vi "Edit_Raw_DF_Header.vi"(0 "Selected files":path[](array[path])) -> ()   [LabVIEW 2013]
uses:
  Controls/File_Selector_Type.ctl
panel:
  in  "Variable names to add by hand":string[](array[string])
  in  "Variable values to add by hand":string[](array[string])
  out "No of Unfound files":i32
  out "Unfound Files":path[](array[path])
  out "File Number":i32
  out "Current case":string
  out "Currently Editting":path
  out "Summary values":string[](array[string])
  in  "New Variable values":string[](array[string])
  in  "Setup Information":i32[](listbox)
  in  "Variable names to Edit":string[](array[string])
  in  "OK":bool
  out "No of Files":i32
  in  "Previous Choice":path
  in  "Search String":string
  in  "At Dialog Prompt for Editting Raw data files":T1
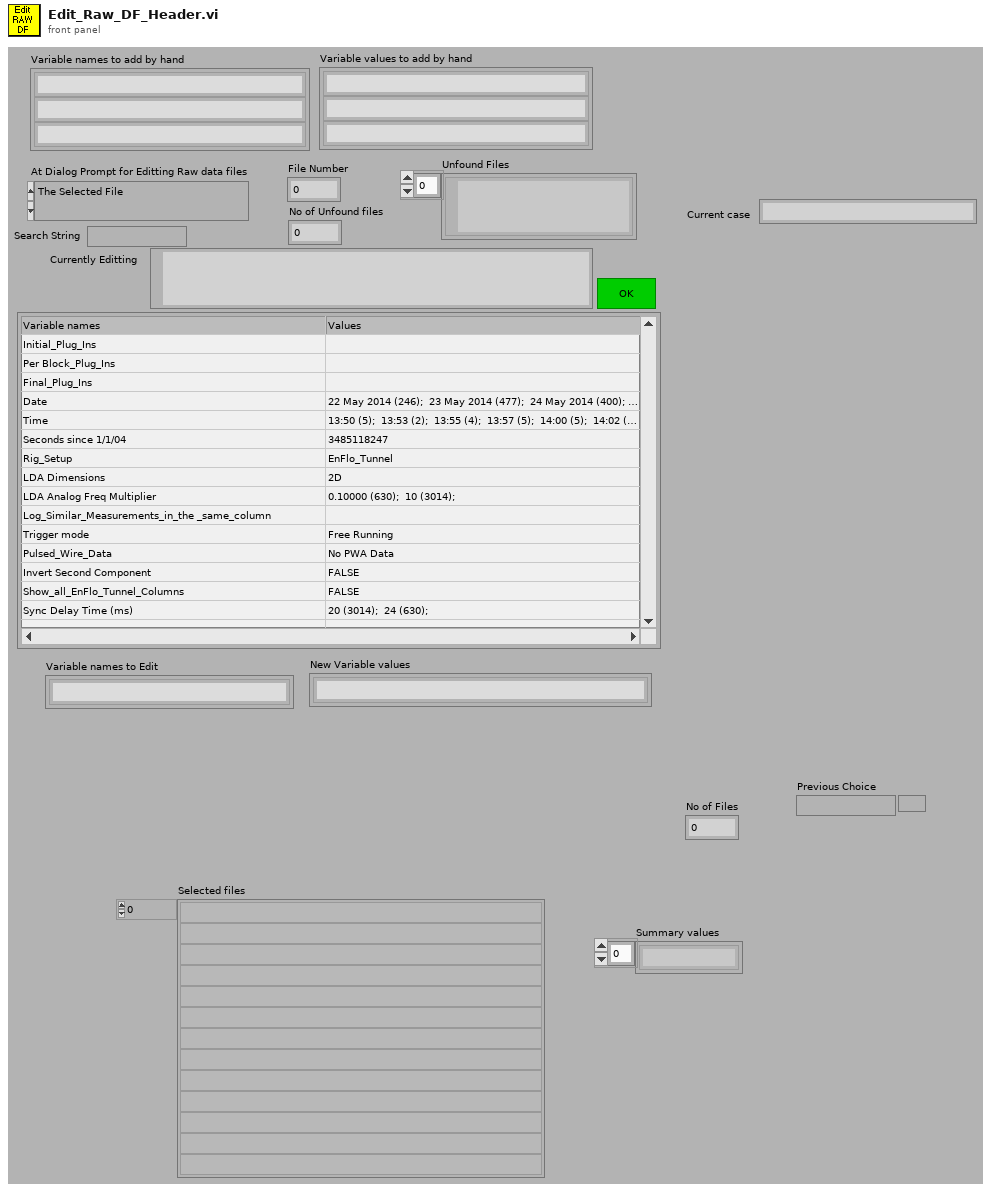
[diagram p1: front panel]
types:
  T1 = typedef "File_Selector_Type.ctl" = enum16{"The Selected File", "The Selected Folder", "Files containing the search string in the selected folder", "All files listed in selected file"}
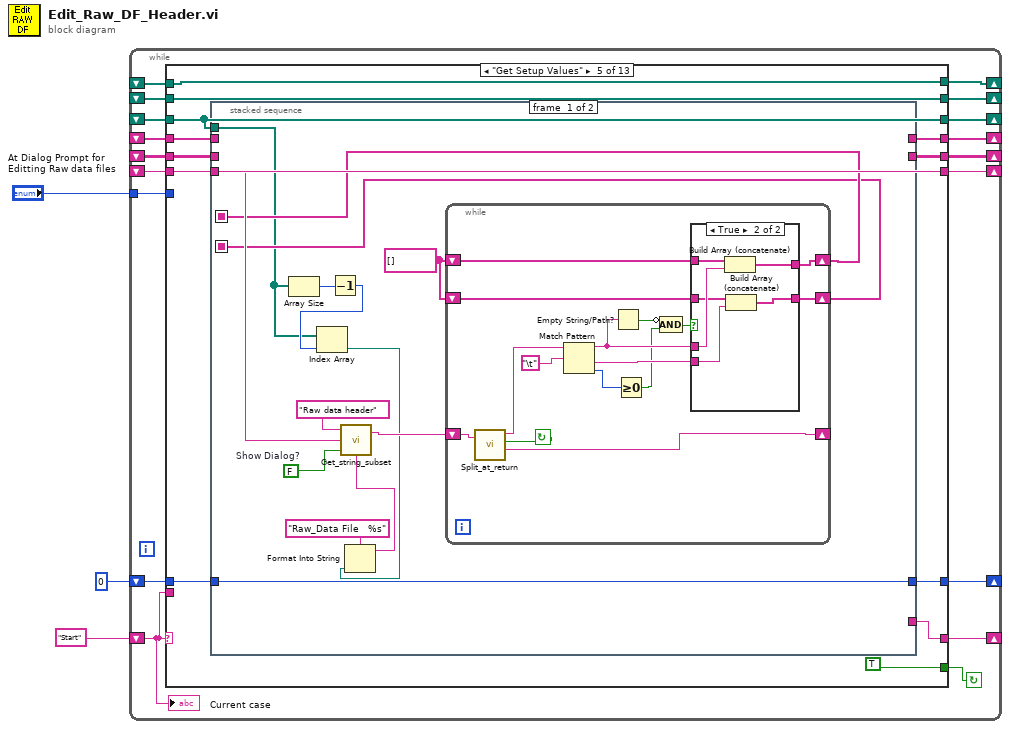
[diagram p0: block diagram]
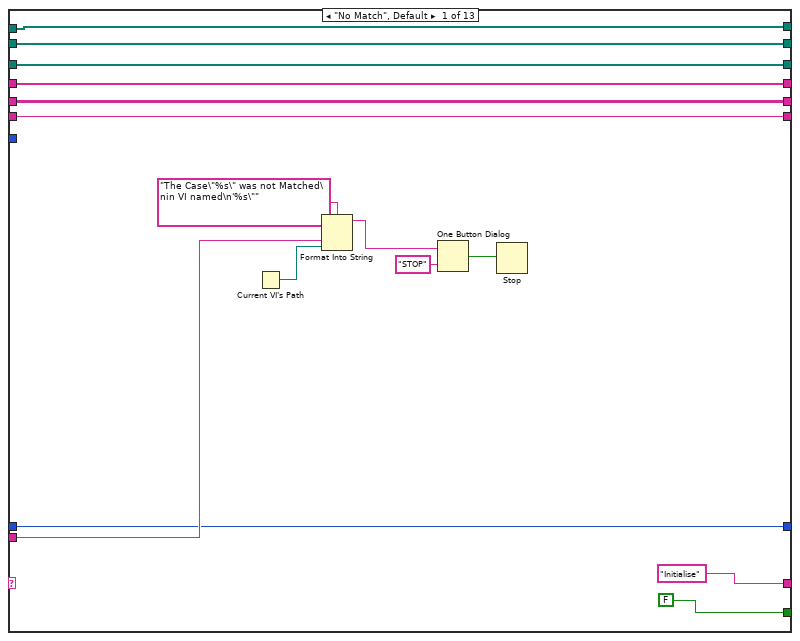
[diagram p2: hidden frame]
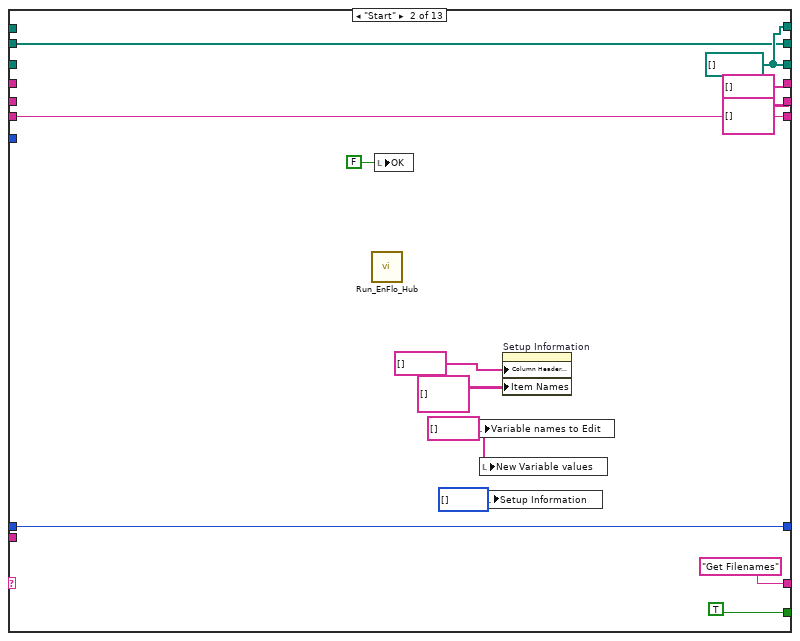
[diagram p3: hidden frame]
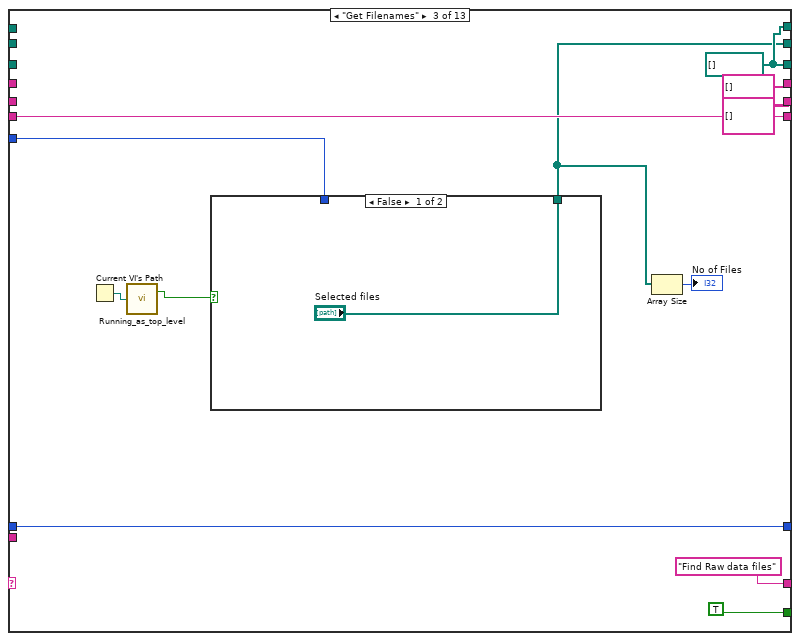
[diagram p4: hidden frame]
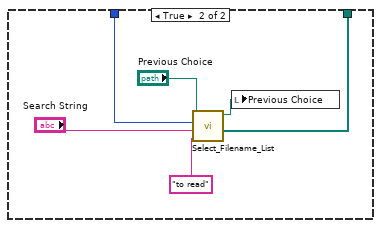
[diagram p5: hidden frame]
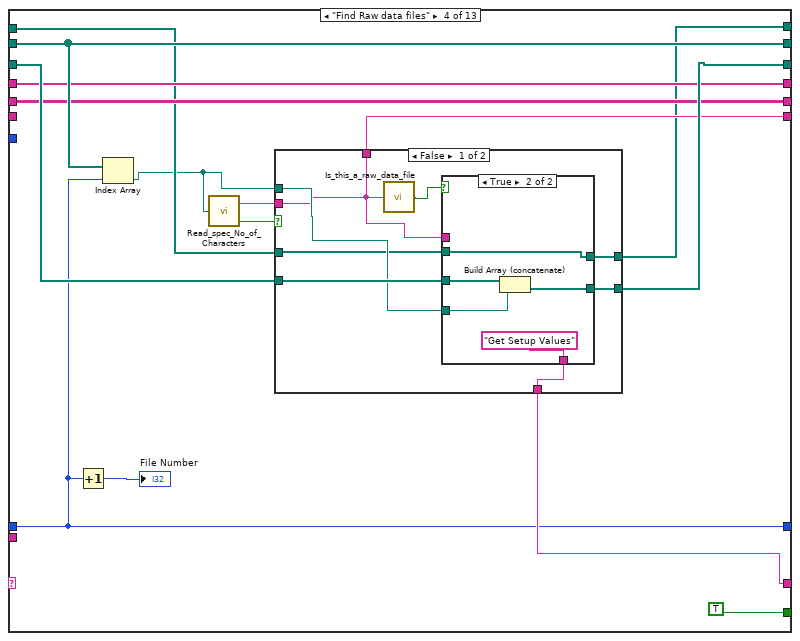
[diagram p6: hidden frame]
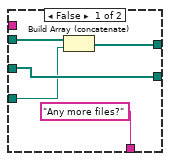
[diagram p7: hidden frame]
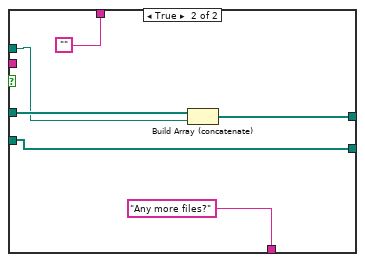
[diagram p8: hidden frame]
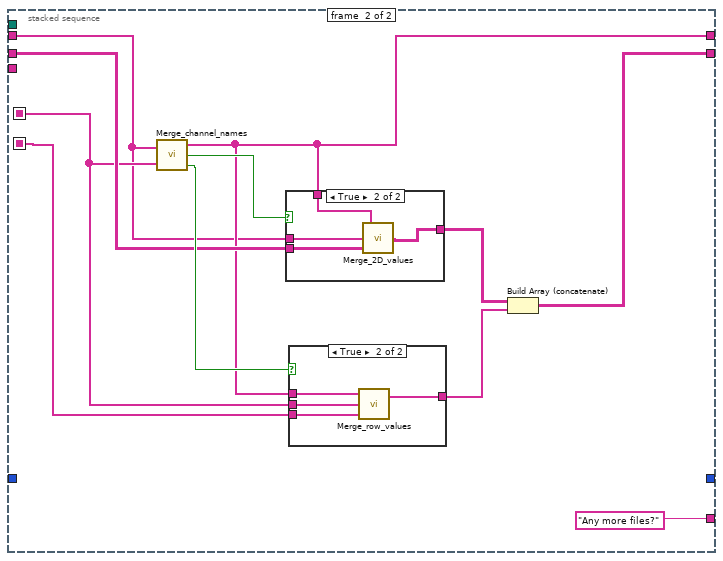
[diagram p10: hidden frame]
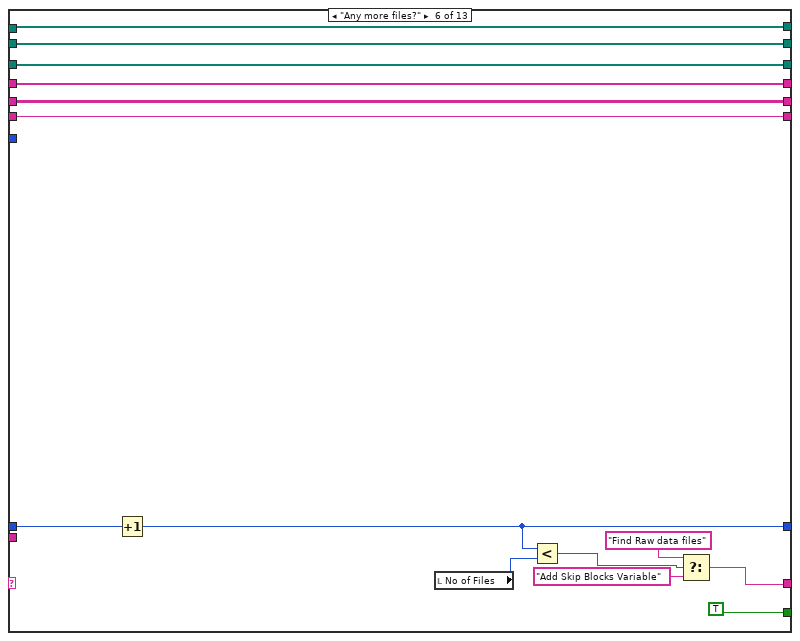
[diagram p13: hidden frame]
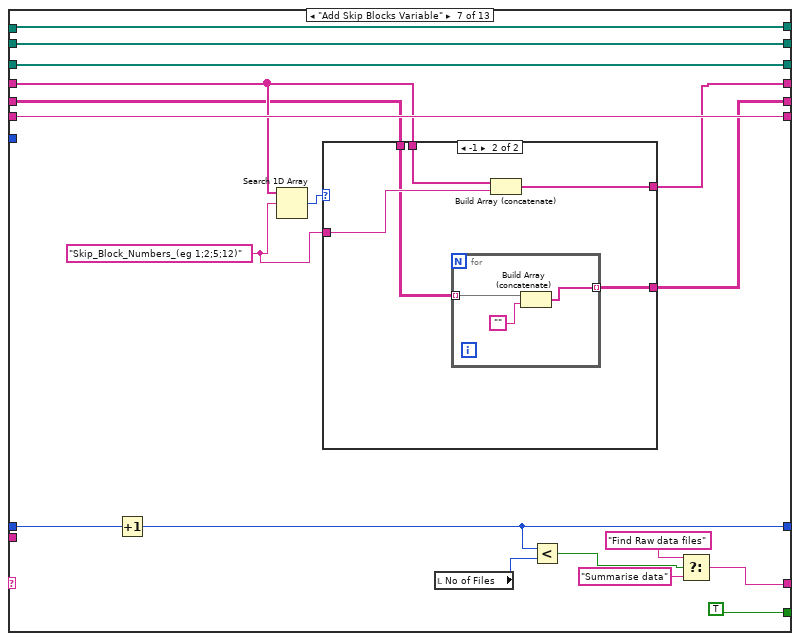
[diagram p14: hidden frame]
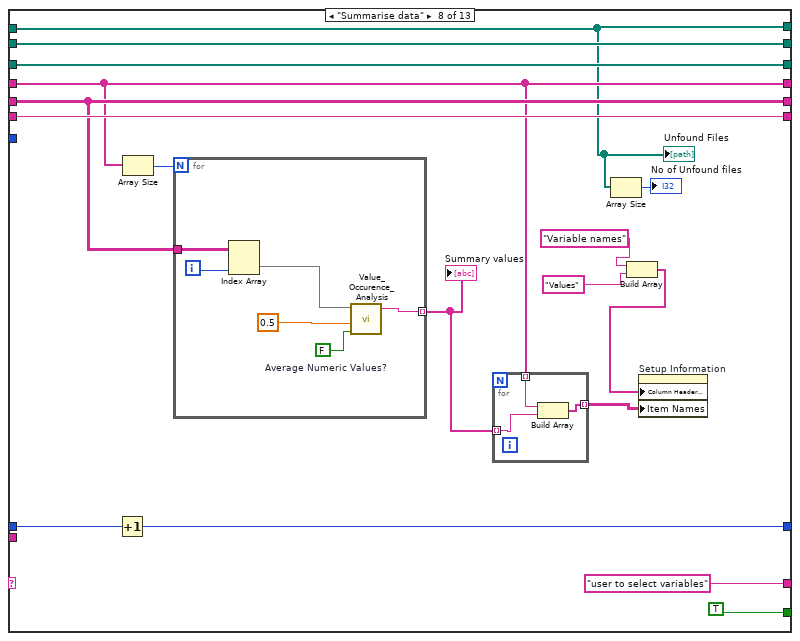
[diagram p16: hidden frame]
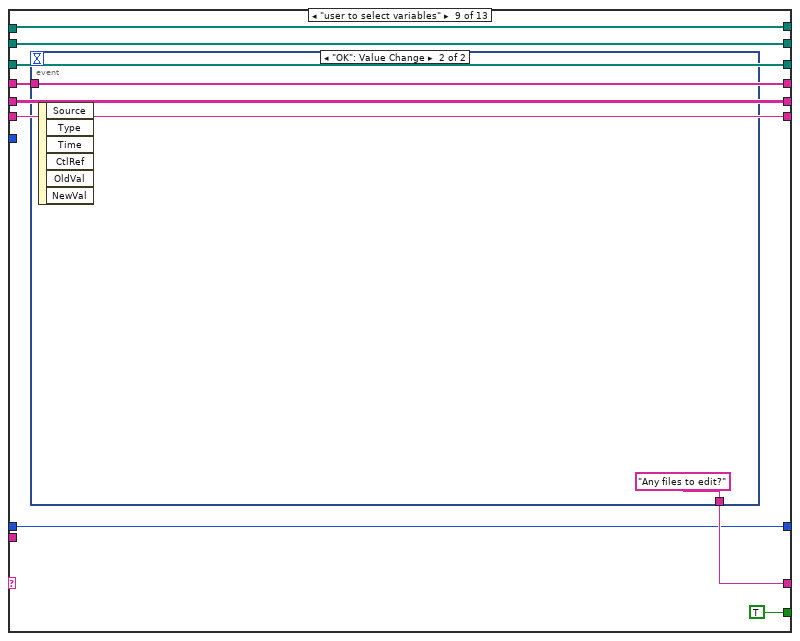
[diagram p17: hidden frame]
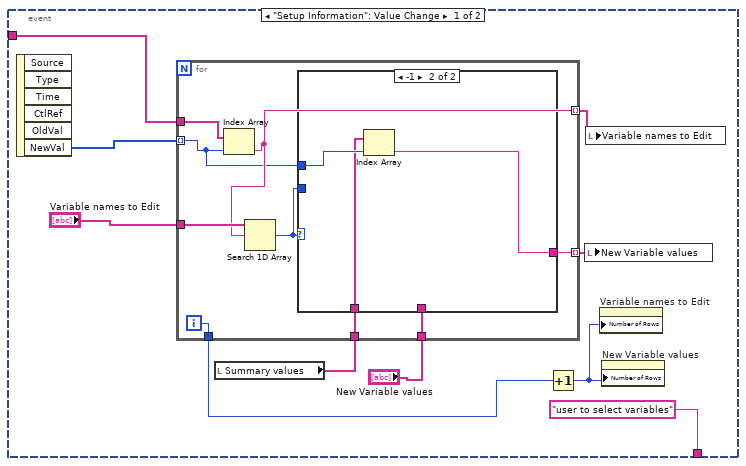
[diagram p18: hidden frame]
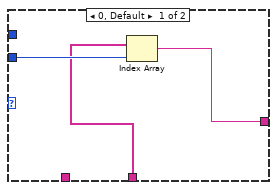
[diagram p19: hidden frame]
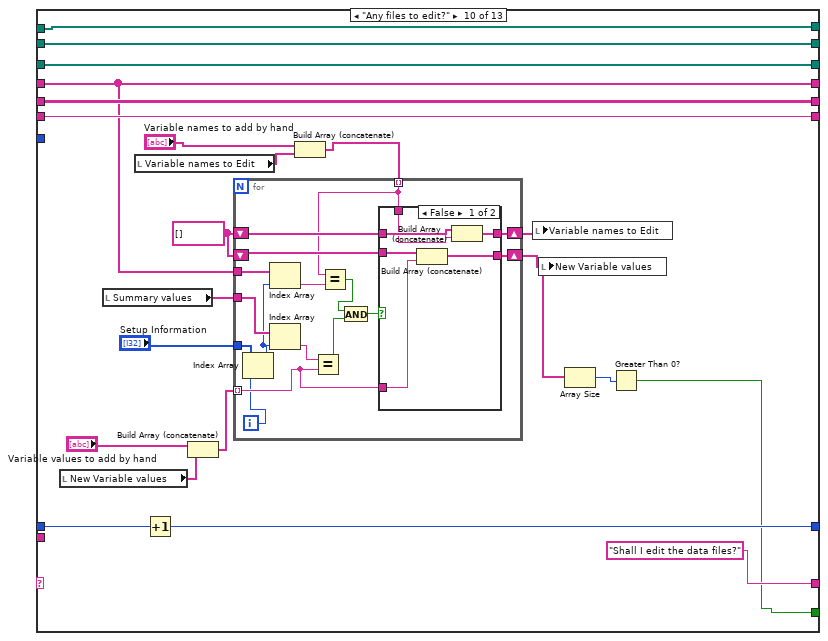
[diagram p20: hidden frame]
diagram:
  n1 = while {
    shift-left: "Start" -> [w19]
    shift-right: [w20] -> _
    shift-right: [w17] -> _
    shift-left: _ -> [w18]
    tunnel: "At Dialog Prompt for Editting Raw data files" -> [w16]
    shift-right: [w7] -> _
    shift-left: 0 -> [w13]
    shift-right: [w15] -> _
    shift-left: _ -> [w14]
    shift-right: [w12] -> _
    shift-left: _ -> [w11]
    shift-right: [w9] -> _
    shift-left: _ -> [w10]
    shift-right: [w8] -> _
    shift-left: _ -> [w6]
    shift-right: [w4] -> _
    shift-left: _ -> [w5]
    stop <- w21 continue-if-true
    n2 = case shown="\"Get Setup Values\"" w19 {
      tunnel: [FALSE TRUE TRUE TRUE TRUE TRUE TRUE TRUE TRUE w289 w328 TRUE ("T button?") FALSE ("T button?")] -> w21
      tunnel: ["Initialise" "Get Filenames" "Find Raw data files" w76 w115 w183 w202 "user to select variables" w248 "Shall I edit the data files?" "Edit Raw data files" "End" "End"] -> w20
      tunnel: w19 -> [w31 _ _ _ _ _ _ _ _ _ _ _ _]
      tunnel: w18 -> [w28 w37 _ w80 w118 w190 w208 w235 w254 w302 w338 w349 w364]
      tunnel: [w28 w37 w50 w80 w118 w190 w208 w235 w254 w302 w338 w349 w364] -> w17
      tunnel: w16 -> [_ _ w60 _ _ _ _ _ _ _ _ _ _]
      tunnel: w14 -> [w27 _ _ w82 w108 w182 w201 w232 w253 w299 w332 w342 w358]
      tunnel: [w27 w38 w53 w81 w108 w182 w201 w232 w253 w299 w332 w342 w358] -> w15
      tunnel: w13 -> [w23 w44 w54 w75 w117 w188 w207 w234 w247 w301 w333 w344 w359]
      tunnel: [w26 string[] [] ("Merged Channels") string[] [] ("Merged Channels") w79 w113 w178 w196 w228 w249 w287 w335 w346 w361] -> w12
      tunnel: w11 -> [w26 _ _ w79 w110 w178 w197 w228 w249 w287 w335 w346 w361]
      tunnel: w10 -> [w25 _ _ w78 w112 w189 w193 w230 w251 w297 w336 w347 w362]
      tunnel: [w25 string[][] [] string[][] [] w78 w111 w189 w192 w230 w251 w297 w336 w347 w362] -> w9
      tunnel: [w24 w47 w57 w77 w114 w181 w200 w231 w252 w298 w337 w348 w363] -> w8
      tunnel: [w23 w44 w54 w75 w116 w187 w206 w233 w247 w300 w333 w344 w359] -> w7
      tunnel: w6 -> [w24 w47 w57 _ w114 w181 w200 w231 w252 w298 w337 w348 w363]
      tunnel: w5 -> [w22 _ _ w74 w109 w179 w198 w221 w246 w288 w327 w339 w354]
      tunnel: [w22 w38 w53 w73 w109 w179 w198 w221 w246 w288 w327 w339 w354] -> w4
      frame "No Match", Default {
        n3 = Current VI's Path() -> (path=w30:path)
        n4 = Format Into String(format string="The Case\"%s\" was not Matched\nin VI named\n'%s\"" ("Format String"), w31, w30) -> (resulting string=w34:string)  [unwired: 2 in, 1 out]
        n5 = One Button Dialog(message=w34, button name ("OK")="STOP") -> (true=w32:bool)
        n6 = Stop(stop? (T)=w32) -> ()
      }
      frame "Start" {
        w43 = string[] [] ("Variable names to Edit")
        w38 = path[] []
        n7 = call "Run_EnFlo_Hub.vi"() -> ()  [unwired: 8 out]
        n8 = local write "OK"(FALSE ("OK")) -> ()
        n9 = local write "Variable names to Edit"(w43) -> ()
        n10 = local write "New Variable values"(w43) -> ()
        n11 = local write "Setup Information"(i32[] [] ("Setup Information")) -> ()
        n12 = property on="Setup Information" class="MCListbox (strict)"("Column Header Strings[]"=string[] [] ("Column Header Strings"), "Item Names"=string[][] []) -> ()  [unwired: 2 in, 2 out]
      }
      frame "Get Filenames" {
        w53 = path[] []
        n13 = Current VI's Path() -> (path=w52:path)
        n14 = call "Running_as_top_level.vi"("Vi path name"=w52) -> ("Top Level"=w51:bool)  [unwired: 1 out]
        n15 = case shown="False" w51 {
          tunnel: w60 -> [_ w68]
          tunnel: ["Selected files" w63] -> w50
          frame False {
          }
          frame True {
            n16 = call "Select_Filename_List.vi"("File Type"="to read", "Search String"="Search String", "At Dialog Prompt Post Process"=w68, "Previous Choice"="Previous Choice") -> ("Selected files"=w63:path[], "Choosen path"=w64:path)  [unwired: 1 in, 2 out]
            n17 = local write "Previous Choice"(w64) -> ()
          }
        }
        n18 = Array Size(array=w50) -> (size(s)=→"No of Files":i32)
      }
      frame "Find Raw data files" {
        n19 = Increment(x=w75) -> (x+1=→"File Number":i32)
        n20 = Index Array(array=w80, index=w75) -> (element=w72:path)
        n21 = call "Read_spec_No_of_Characters.vi"("Filename"=w72) -> ("character string"=w70:string, "Error?"=w71:bool)
        n22 = case shown="False" w71 {
          tunnel: w82 -> [w91 w107]
          tunnel: [w90 w107] -> w81
          tunnel: w72 -> [w88 w103]
          tunnel: [w84 ""] -> w77
          tunnel: [w87 "Any more files?"] -> w76
          tunnel: w74 -> [w86 w104]
          tunnel: [w85 w102] -> w73
          tunnel: w70 -> [w84 _]
          frame False {
            n23 = call "Is_this_a_raw_data_file.vi"("character string"=w84) -> ("Raw Dat File?"=w89:bool)  [unwired: 2 out]
            n24 = case shown="True" w89 {
              tunnel: w91 -> [w96 w101]
              tunnel: w88 -> [w92 w100]
              tunnel: [w96 w99] -> w90
              tunnel: w84 -> [_ _]
              tunnel: ["Any more files?" "Get Setup Values"] -> w87
              tunnel: w86 -> [w94 w97]
              tunnel: [w93 w97] -> w85
              frame False {
                n25 = Build Array (concatenate)(w94, w92) -> (w93:path[])
              }
              frame True {
                n26 = Build Array (concatenate)(w101, w100) -> (w99:path[])
              }
            }
          }
          frame True {
            n27 = Build Array (concatenate)(w104, w103) -> (w102:path[])
          }
        }
      }
      frame "Get Setup Values" {
        n28 = stacked-sequence {
          seq-local: [w127 _] -> [_ w158]
          seq-local: [w126 _] -> [_ w160]
          tunnel: w117 -> [w130 _]
          tunnel: [w130 _] -> w116
          tunnel: [_ "Any more files?"] -> w115
          tunnel: w114 -> [w131 _]
          tunnel: w110 -> [_ w157]
          tunnel: [_ w161] -> w113
          tunnel: w112 -> [_ w165]
          tunnel: [_ w162] -> w111
          tunnel: w108 -> [w121 _]
          frame #0 {
            w128 = string[] []
            w133 = FALSE  # Show Dialog?
            n29 = Array Size(array=w121) -> (size(s)=w123:i32)
            n30 = Decrement(x=w123) -> (x-1=w122:i32)
            n31 = Index Array(array=w121, index=w122) -> (element=w120:path)
            n32 = Format Into String(format string="Raw_Data File   %s", w120) -> (resulting string=w124:string)  [unwired: 2 in, 1 out]
            n33 = call "Get_string_subset.vi"("String Name"=w124, "Show Dialog?"=w133, "String to split"=w131, "File Label"="Raw data header") -> ("Output string"=w129:string)  [unwired: 1 out]
            n34 = while {
              shift-right: [w147] -> _
              shift-left: w129 -> [w148]
              shift-right: [w141] -> w127
              shift-left: w128 -> [w142]
              shift-right: [w139] -> w126
              shift-left: w128 -> [w140]
              stop <- w146 continue-if-true
              n35 = call "Split_at_return.vi"("String"=w148) -> ("before substring"=w144:string, "Matched?"=w146:bool, "after substring"=w147:string)  [unwired: 1 in, 1 out]
              n36 = Match Pattern(string=w144, regular expression="\t") -> (before substring=w137:string, after substring=w138:string, offset past match=w143:i32)  [unwired: 2 out]
              n37 = Empty String/Path?(string/path=w137) -> (empty?=w136:bool)
              n38 = Greater Or Equal To 0?(x=w143) -> (x >= 0?=w134:bool)
              n39 = Compound Arithmetic op=AND(invert w136, w134) -> (w135:bool)
              n40 = case shown="True" w135 {
                tunnel: w142 -> [w150 w156]
                tunnel: w137 -> [_ w155]
                tunnel: [w150 w154] -> w141
                tunnel: w140 -> [w149 w153]
                tunnel: [w149 w152] -> w139
                tunnel: w138 -> [_ w151]
                frame False {
                }
                frame True {
                  n41 = Build Array (concatenate)(w156, w155) -> (w154:string[])
                  n42 = Build Array (concatenate)(w153, w151) -> (w152:string[])
                }
              }
            }
          }
          frame #1 {
            n43 = call "Merge_channel_names.vi"("Preferred Channel array"=w157, "Channel array"=w158) -> ("Merged Channels"=w161:string[], "Preferred Channels Changed?"=w166:bool, "Channel Array Changed?"=w167:bool)
            n44 = case shown="True" w166 {
              tunnel: w165 -> [w173 w175]
              tunnel: w157 -> [_ w177]
              tunnel: [w173 w174] -> w164
              tunnel: w161 -> [_ w176]
              frame False {
              }
              frame True {
                n45 = call "Merge_2D_values.vi"("Values In"=w175, "Present Channels"=w177, "Desired Channels"=w176) -> ("Values Out"=w174:string[][])
              }
            }
            n46 = case shown="True" w167 {
              tunnel: [w168 w172] -> w163
              tunnel: w161 -> [_ w171]
              tunnel: w158 -> [_ w170]
              tunnel: w160 -> [w168 w169]
              frame False {
              }
              frame True {
                n47 = call "Merge_row_values.vi"("Present Row values"=w169, "Present Channels"=w170, "Desired Channels"=w171) -> ("Desired Row values"=w172:string[])  [unwired: 1 out]
              }
            }
            n48 = Build Array (concatenate)(w164, w163) -> (w162:string[][])
          }
        }
      }
      frame "Any more files?" {
        n49 = Increment(x=w188) -> (x+1=w187:i32)
        n50 = local read "No of Files"() -> (w186:i32)
        n51 = Less?(x=w187, y=w186) -> (x < y?=w185:bool)
        n52 = Select(t="Find Raw data files", s=w185, f="Add Skip Blocks Variable") -> (s? t:f=w183:string)
      }
      frame "Add Skip Blocks Variable" {
        w195 = "Skip_Block_Numbers_(eg 1;2;5;12)" ("Variable name")
        n53 = Increment(x=w207) -> (x+1=w206:i32)
        n54 = Search 1D Array(1D array=w197, element=w195) -> (index of element=w194:i32)  [unwired: 1 out]
        n55 = case shown="-1" w194 {
          tunnel: w197 -> [w211 w216]
          tunnel: w195 -> [_ w215]
          tunnel: [w211 w214] -> w196
          tunnel: w193 -> [w210 w213]
          tunnel: [w210 w212] -> w192
          frame 0, Default {
          }
          frame -1 {
            n56 = for {
              tunnel: w213 -> [w218] mode=indexing
              tunnel: [w217] -> w212 mode=indexing
              n57 = Build Array (concatenate)(w218, "") -> (w217:string[])
            }
            n58 = Build Array (concatenate)(w216, w215) -> (w214:string[])
          }
        }
        n59 = local read "No of Files"() -> (w205:i32)
        n60 = Less?(x=w206, y=w205) -> (x < y?=w204:bool)
        n61 = Select(t="Find Raw data files", s=w204, f="Summarise data") -> (s? t:f=w202:string)
      }
      frame "Summarise data" {
        n62 = Increment(x=w234) -> (x+1=w233:i32)
        n63 = Array Size(array=w228) -> (size(s)=w229:i32)
        n64 = for {
          N: w229 -> [_]
          tunnel: w230 -> [w244]
          tunnel: [w240] -> w227 mode=indexing
          i -> [w245]
          w241 = FALSE  # Average Numeric Values?
          n65 = Index Array(array=w244, index (col)=w245) -> (element=w243:string[])  [unwired: 1 in]
          n66 = call "Value_Occurence_Analysis.vi"("Average Numeric Values?"=w241, "Tolerance"=0.5, "String Array"=w243) -> ("Output String"=w240:string)  [unwired: 1 in, 2 out]
        }
        "Summary values" <- w227
        n67 = for {
          tunnel: w228 -> [w238] mode=indexing
          tunnel: w227 -> [w239] mode=indexing
          tunnel: [w237] -> w223 mode=indexing
          n68 = Build Array(w238, w239) -> (w237:string[])
        }
        n69 = Array Size(array=w221) -> (size(s)=→"No of Unfound files":i32)
        n70 = Build Array("Variable names", "Values") -> (w222:string[])
        n71 = property on="Setup Information" class="MCListbox (strict)"("Column Header Strings[]"=w222, "Item Names"=w223) -> ()  [unwired: 2 in, 2 out]
        "Unfound Files" <- w221
      }
      frame "user to select variables" {
        n72 = event shown="[1] \"OK\": Value Change" {
          selector: _ -> [_ _]
          dyn-events: _ -> [_ _]
          timeout: _ -> [_ _]
          tunnel: w249 -> [w263 _]
          tunnel: ["user to select variables" "Any files to edit?"] -> w248
          event "Setup Information": Value Change {
            n73 = event-data() -> ("NewVal"=w264:i32[])  [unwired: 6 out]
            n74 = local read "Summary values"() -> (w262:string[])
            n75 = for {
              tunnel: w264 -> [w270] mode=indexing
              tunnel: w263 -> [w273]
              tunnel: "Variable names to Edit" -> [w272]
              tunnel: [w271] -> w256 mode=indexing
              tunnel: w262 -> [w269]
              tunnel: [w268] -> w261 mode=indexing
              tunnel: "New Variable values" -> [w266]
              tunnel: [w265] -> w258
              i -> [w265]
              n76 = Index Array(array=w273, index=w270) -> (element=w271:string)
              n77 = Search 1D Array(1D array=w272, element=w271) -> (index of element=w267:i32)  [unwired: 1 out]
              n78 = case shown="-1" w267 {
                tunnel: w270 -> [_ w279]
                tunnel: w269 -> [_ w278]
                tunnel: [w274 w277] -> w268
                tunnel: w267 -> [w276 _]
                tunnel: w266 -> [w275 _]
                frame 0, Default {
                  n79 = Index Array(array=w275, index=w276) -> (element=w274:string)
                }
                frame -1 {
                  n80 = Index Array(array=w278, index=w279) -> (element=w277:string)
                }
              }
            }
            n81 = Increment(x=w258) -> (x+1=w257:i32)
            n82 = local write "New Variable values"(w261) -> ()
            n83 = local write "Variable names to Edit"(w256) -> ()
            n84 = property on="Variable names to Edit" class="Arr (strict)"("Number of Rows"=w257) -> ()  [unwired: 2 in, 2 out]
            n85 = property on="New Variable values" class="Arr (strict)"("Number of Rows"=w257) -> ()  [unwired: 2 in, 2 out]
          }
          event "OK": Value Change {
            n86 = event-data() -> ()  [unwired: 7 out]
          }
        }
      }
      frame "Any files to edit?" {
        w293 = string[] []
        n87 = local read "New Variable values"() -> (w286:string[])
        n88 = local read "Summary values"() -> (w294:string[])
        n89 = local read "Variable names to Edit"() -> (w283:string[])
        n90 = Increment(x=w301) -> (x+1=w300:i32)
        n91 = Build Array (concatenate)("Variable values to add by hand", w286) -> (w284:string[])
        n92 = Build Array (concatenate)("Variable names to add by hand", w283) -> (w281:string[])
        n93 = for {
          tunnel: "Setup Information" -> [w305]
          tunnel: w294 -> [w318]
          tunnel: w284 -> [w312] mode=indexing
          shift-right: [w315] -> w292
          shift-left: w293 -> [w316]
          shift-right: [w313] -> w291
          shift-left: w293 -> [w314]
          tunnel: w281 -> [w310] mode=indexing
          tunnel: w287 -> [w311]
          i -> [w304]
          n94 = Index Array(array=w305, index=w304) -> (element=w303:i32)
          n95 = Index Array(array=w311, index=w303) -> (element=w309:string)
          n96 = Index Array(array=w318, index=w303) -> (element=w317:string)
          n97 = Equal?(x=w317, y=w312) -> (x = y?=w308:bool)
          n98 = Equal?(x=w310, y=w309) -> (x = y?=w307:bool)
          n99 = And(x=w307, y=w308) -> (x .and. y?=w306:bool)
          n100 = case shown="False" w306 {
            tunnel: w316 -> [w324 w326]
            tunnel: [w323 w326] -> w315
            tunnel: w314 -> [w322 w325]
            tunnel: [w321 w325] -> w313
            tunnel: w312 -> [w320 _]
            tunnel: w310 -> [w319 _]
            frame False {
              n101 = Build Array (concatenate)(w322, w320) -> (w321:string[])
              n102 = Build Array (concatenate)(w324, w319) -> (w323:string[])
            }
            frame True {
            }
          }
        }
        n103 = local write "Variable names to Edit"(w292) -> ()
        n104 = local write "New Variable values"(w291) -> ()
        n105 = Array Size(array=w291) -> (size(s)=w290:i32)
        n106 = Greater Than 0?(x=w290) -> (x > 0?=w289:bool)
      }
      frame "Shall I edit the data files?" {
        n107 = Array Size(array=w332) -> (size(s)=w331:i32)
        n108 = Format Into String(format string="Do you want to edit these raw data header values in %d Raw Data Files?" ("message"), w331) -> (resulting string=w329:string)  [unwired: 2 in, 1 out]
        n109 = Two Button Dialog(message=w329) -> (T button?=w328:bool)  [unwired: 2 out]
        n110 = property on="Currently Editting" class="Path"("Visible"=w328) -> ()  [unwired: 2 in, 2 out]
      }
      frame "Edit Raw data files" {
        n111 = local read "Variable names to Edit"() -> (w343:string[])
        n112 = local read "New Variable values"() -> (w340:string[])
        n113 = for {
          tunnel: w343 -> [w353]
          tunnel: w340 -> [w350]
          tunnel: w342 -> [w351] mode=indexing
          w352 = TRUE  # Edit Raw Data Header Info
          n114 = call "Edit_Raw_DF_Remote.vi"("Edit Raw Data Header Info"=w352, "New Values In"=w350, "New Chs In"=w353, "Current Filename"=w351) -> ()  [unwired: 4 out]
          "Currently Editting" <- w351
        }
      }
      frame "End" {
        n115 = property on="Currently Editting" class="Path"("Visible"=FALSE) -> ()  [unwired: 2 in, 2 out]
        n116 = local write "OK"(FALSE ("OK")) -> ()
      }
    }
    "Current case" <- w19
  }
